vi "Begin.vi"() -> (0 "Error out":errorcluster)   [LabVIEW 2015]
doc: "Called before other user functions, this VI is expected to open initial I/O refnums, load in file data, and do all program initialization. Notice that the <B>error out</B> terminal is simply used for data flow. Wiring it to other structures or subVIs ensures that this VI runs first."
uses:
  <vilib>/Rock Robotics/WPI/Joystick/WPI_JoystickDeviceEnum.ctl
  <vilib>/Rock Robotics/WPI/Solenoid/WPI_SolenoidChannel.ctl
  <vilib>/Rock Robotics/WPI/CAN/TalonSRX/WPI_CANTalonSRX_APIControlMode.ctl
  <vilib>/Rock Robotics/SystemInterfaces/DIO/FPGA_DIOPWMChannel.ctl
  <vilib>/Rock Robotics/SystemInterfaces/AI/FPGA_AIGyroChannel.ctl
  <vilib>/Rock Robotics/SystemInterfaces/DIO/FPGA_DIOChannel.ctl
  <vilib>/Rock Robotics/WPI/CAN/TalonSRX/WPI_CANTalonSRX_APIFeedbackSelect.ctl
  <vilib>/Rock Robotics/WPI/Solenoid/WPI_SolenoidValue.ctl
  <vilib>/Rock Robotics/SystemInterfaces/i2clib/i2c_bus.ctl
  <vilib>/Rock Robotics/WPI/MotorControl/WPI_MotorControlOpenCANTalonSRX.vi
  <vilib>/Rock Robotics/WPI/Solenoid/WPI_SolenoidOpenDouble.vi
  <vilib>/Rock Robotics/WPI/Gyro/WPI_GyroAnalogOpen.vi
  <vilib>/Rock Robotics/WPI/Switch/WPI_SwitchOpenLimit.vi
  <vilib>/Rock Robotics/WPI/MotorControl/WPI_MotorControlOpen VictorSP.vi
  Global Variables/Temp Variables.vi
  <vilib>/Rock Robotics/WPI/Solenoid/WPI_SolenoidOpenSingle.vi
  <vilib>/Rock Robotics/WPI/Solenoid/WPI_SolenoidSetEnum.vi
  Global Variables/refnum names.vi
  Global Variables/Calibrations.vi
  <vilib>/Rock Robotics/SystemInterfaces/AI/FPGA_AIChannel.ctl
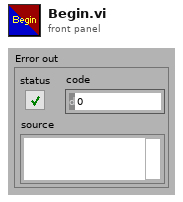
[diagram p1: front panel]
types:
  T1 = typedef "i2c_bus.ctl" = enum16{"I2C On-Board", "I2C MXP", "Invalid"}
  T2 = enum8{"ConfigMode", "AccOnly", "MagOnly", "GyroOnly", "AccMag", "AccGyro", "MagGyro", "AMG", "IMU", "Compass", "M4G", "NDOF_FMC_OFF", "NDOF"}
  T3 = enum32{"P0", "P1", "P2", "P3", "P4", "P5", "P6", "P7"}
  T4 = typedef "WPI_SolenoidChannel.ctl" = enum8{"Solenoid 0", "Solenoid 1", "Solenoid 2", "Solenoid 3", "Solenoid 4", "Solenoid 5", "Solenoid 6", "Solenoid 7", "Invalid"}
  T5 = typedef "WPI_SolenoidValue.ctl" = enum16{"Off", "On", "Forward", "Reverse"}
  T6 = typedef "WPI_CANTalonSRX_APIControlMode.ctl" = enum8{"Percent VBus", "Speed", "Position", "Slave", "Unchanged / Invalid", "Voltage Compensation", "Current", "Motion Profile"}
  T7 = typedef "FPGA_DIOChannel.ctl" = enum8{"DIO 0", "DIO 1", "DIO 2", "DIO 3", "DIO 4", "DIO 5", "DIO 6", "DIO 7", "DIO 8", "DIO 9", "DIO MXP 0", "DIO MXP 1", "DIO MXP 2", "DIO MXP 3", "DIO MXP 4", "DIO MXP 5", "DIO MXP 6", "DIO MXP 7", "DIO MXP 8", "DIO MXP 9", "DIO MXP 10", "DIO MXP 11", "DIO MXP 12", "DIO MXP 13", "DIO MXP 14", "DIO MXP 15", "Invalid"}
  T8 = typedef "WPI_JoystickDeviceEnum.ctl" = enum16{"USB 0", "USB 1", "USB 2", "USB 3", "USB 4", "USB 5"}
  T9 = typedef "WPI_CANTalonSRX_APIFeedbackSelect.ctl" = enum16{"Digital Quadrature Encoder", "Analog Potentiometer", "Analog Encoder", "Count on Quad-A (Rising-Edge)", "Count on Quad-A (Falling-Edge)", "CTR Magnetic Enc (Absolute)", "CTR Magnetic Enc (Relative)", "Pulse Width"}
  T10 = typedef "FPGA_AIGyroChannel.ctl" = enum8{"AI 0", "AI 1", "Invalid"}
  T11 = typedef "FPGA_DIOPWMChannel.ctl" = enum8{"PWM 0", "PWM 1", "PWM 2", "PWM 3", "PWM 4", "PWM 5", "PWM 6", "PWM 7", "PWM 8", "PWM 9", "PWM MXP 0", "PWM MXP 1", "PWM MXP 2", "PWM MXP 3", "PWM MXP 4", "PWM MXP 5", "PWM MXP 6", "PWM MXP 7", "PWM MXP 8", "PWM MXP 9", "Invalid"}
  T12 = typedef "FPGA_AIChannel.ctl" = enum8{"AI 0", "AI 1", "AI 2", "AI 3", "AI MXP 0", "AI MXP 1", "AI MXP 2", "AI MXP 3", "Invalid"}
  T13 = typedef "WPI_MotorControlDeviceRef.ctl" = cluster{"DeviceStatus":errorcluster, "Type":T14, "PWM":cluster{"PWM Channel":T11, "DeadBand":T15}, "CAN":cluster{"Device Number":u8, "Control Mode":T16, "Semaphore":T17, "Max Vout":dbl, "TalonSRX Control Mode":T6}, "Invert":bool}
  T14 = typedef "WPI_MotorControlType.ctl" = enum16{"PWM", "CAN", "CANTalonSRX"}
  T15 = typedef "WPI_PWMDeadband.ctl" = cluster{"Name":string, "maxPositivePwm":i32, "minPositivePwm":i32, "centerPwm":i32, "maxNegativePwm":i32, "minNegativePwm":i32, "angularRange":u16}
  T16 = typedef "WPI_CANJaguar_ControlMode.ctl" = enum8{"Percent VBus", "Current", "Speed", "Position", "Voltage"}
  T17 = typedef "Semaphore RefNum" = refnum<k1>
  T18 = typedef "WPI_I2CDevRef.ctl" = cluster{"DevStatus":errorcluster, "Device Address":u8, "Handle":i32, "I2C Bus":T1}
  T19 = typedef "WPI_PotentiometerDevRef.ctl" = cluster{"DevStatus":errorcluster, "Analog Channel":T12, "Invert Output":bool}
  T20 = typedef "WPI_SolenoidDevRef.ctl" = cluster{"DevStatus":errorcluster, "Pneumatics Control Module":u8, "Forward Solenoid Channel":T4, "Reverse Solenoid Channel":T4}
  T21 = typedef "WPI_GyroDevRef.ctl" = cluster{"DevStatus":errorcluster, "Analog Channel":T12, "Offset":dbl, "Gain (VoltsPerDegree/Second)":dbl, "Gyro Type":enum16{"Analog", "XRS450"}, "Handle":i32, "SPI Bus":T22, "Device Found":bool, "Sample Rate":dbl, "Calibrate On Open":bool}
  T22 = typedef "spi_bus.ctl" = enum16{"SPI On-Board, CS0", "SPI On-Board, CS1", "SPI On-Board, CS2", "SPI On-Board, CS3", "SPI MXP", "Invalid"}
  T23 = typedef "WPI_SwitchDevRef.ctl" = cluster{"DevStatus":errorcluster, "DIO Channel":T7, "CntIndex":T24, "Normally Closed":bool}
  T24 = typedef "FPGA_CounterCtrSystemIndex.ctl" = enum8{"Ctr 0", "Ctr 1", "Ctr 2", "Ctr 3", "Ctr 4", "Ctr 5", "Ctr 6", "Ctr 7", "Invalid"}
  T25 = typedef "WPI_DigitalInputDevRef.ctl" = cluster{"DevStatus":errorcluster, "DIO Channel":T7}
  T26 = typedef "WPI_JoystickDevRef.ctl" = cluster{"Device":T8}
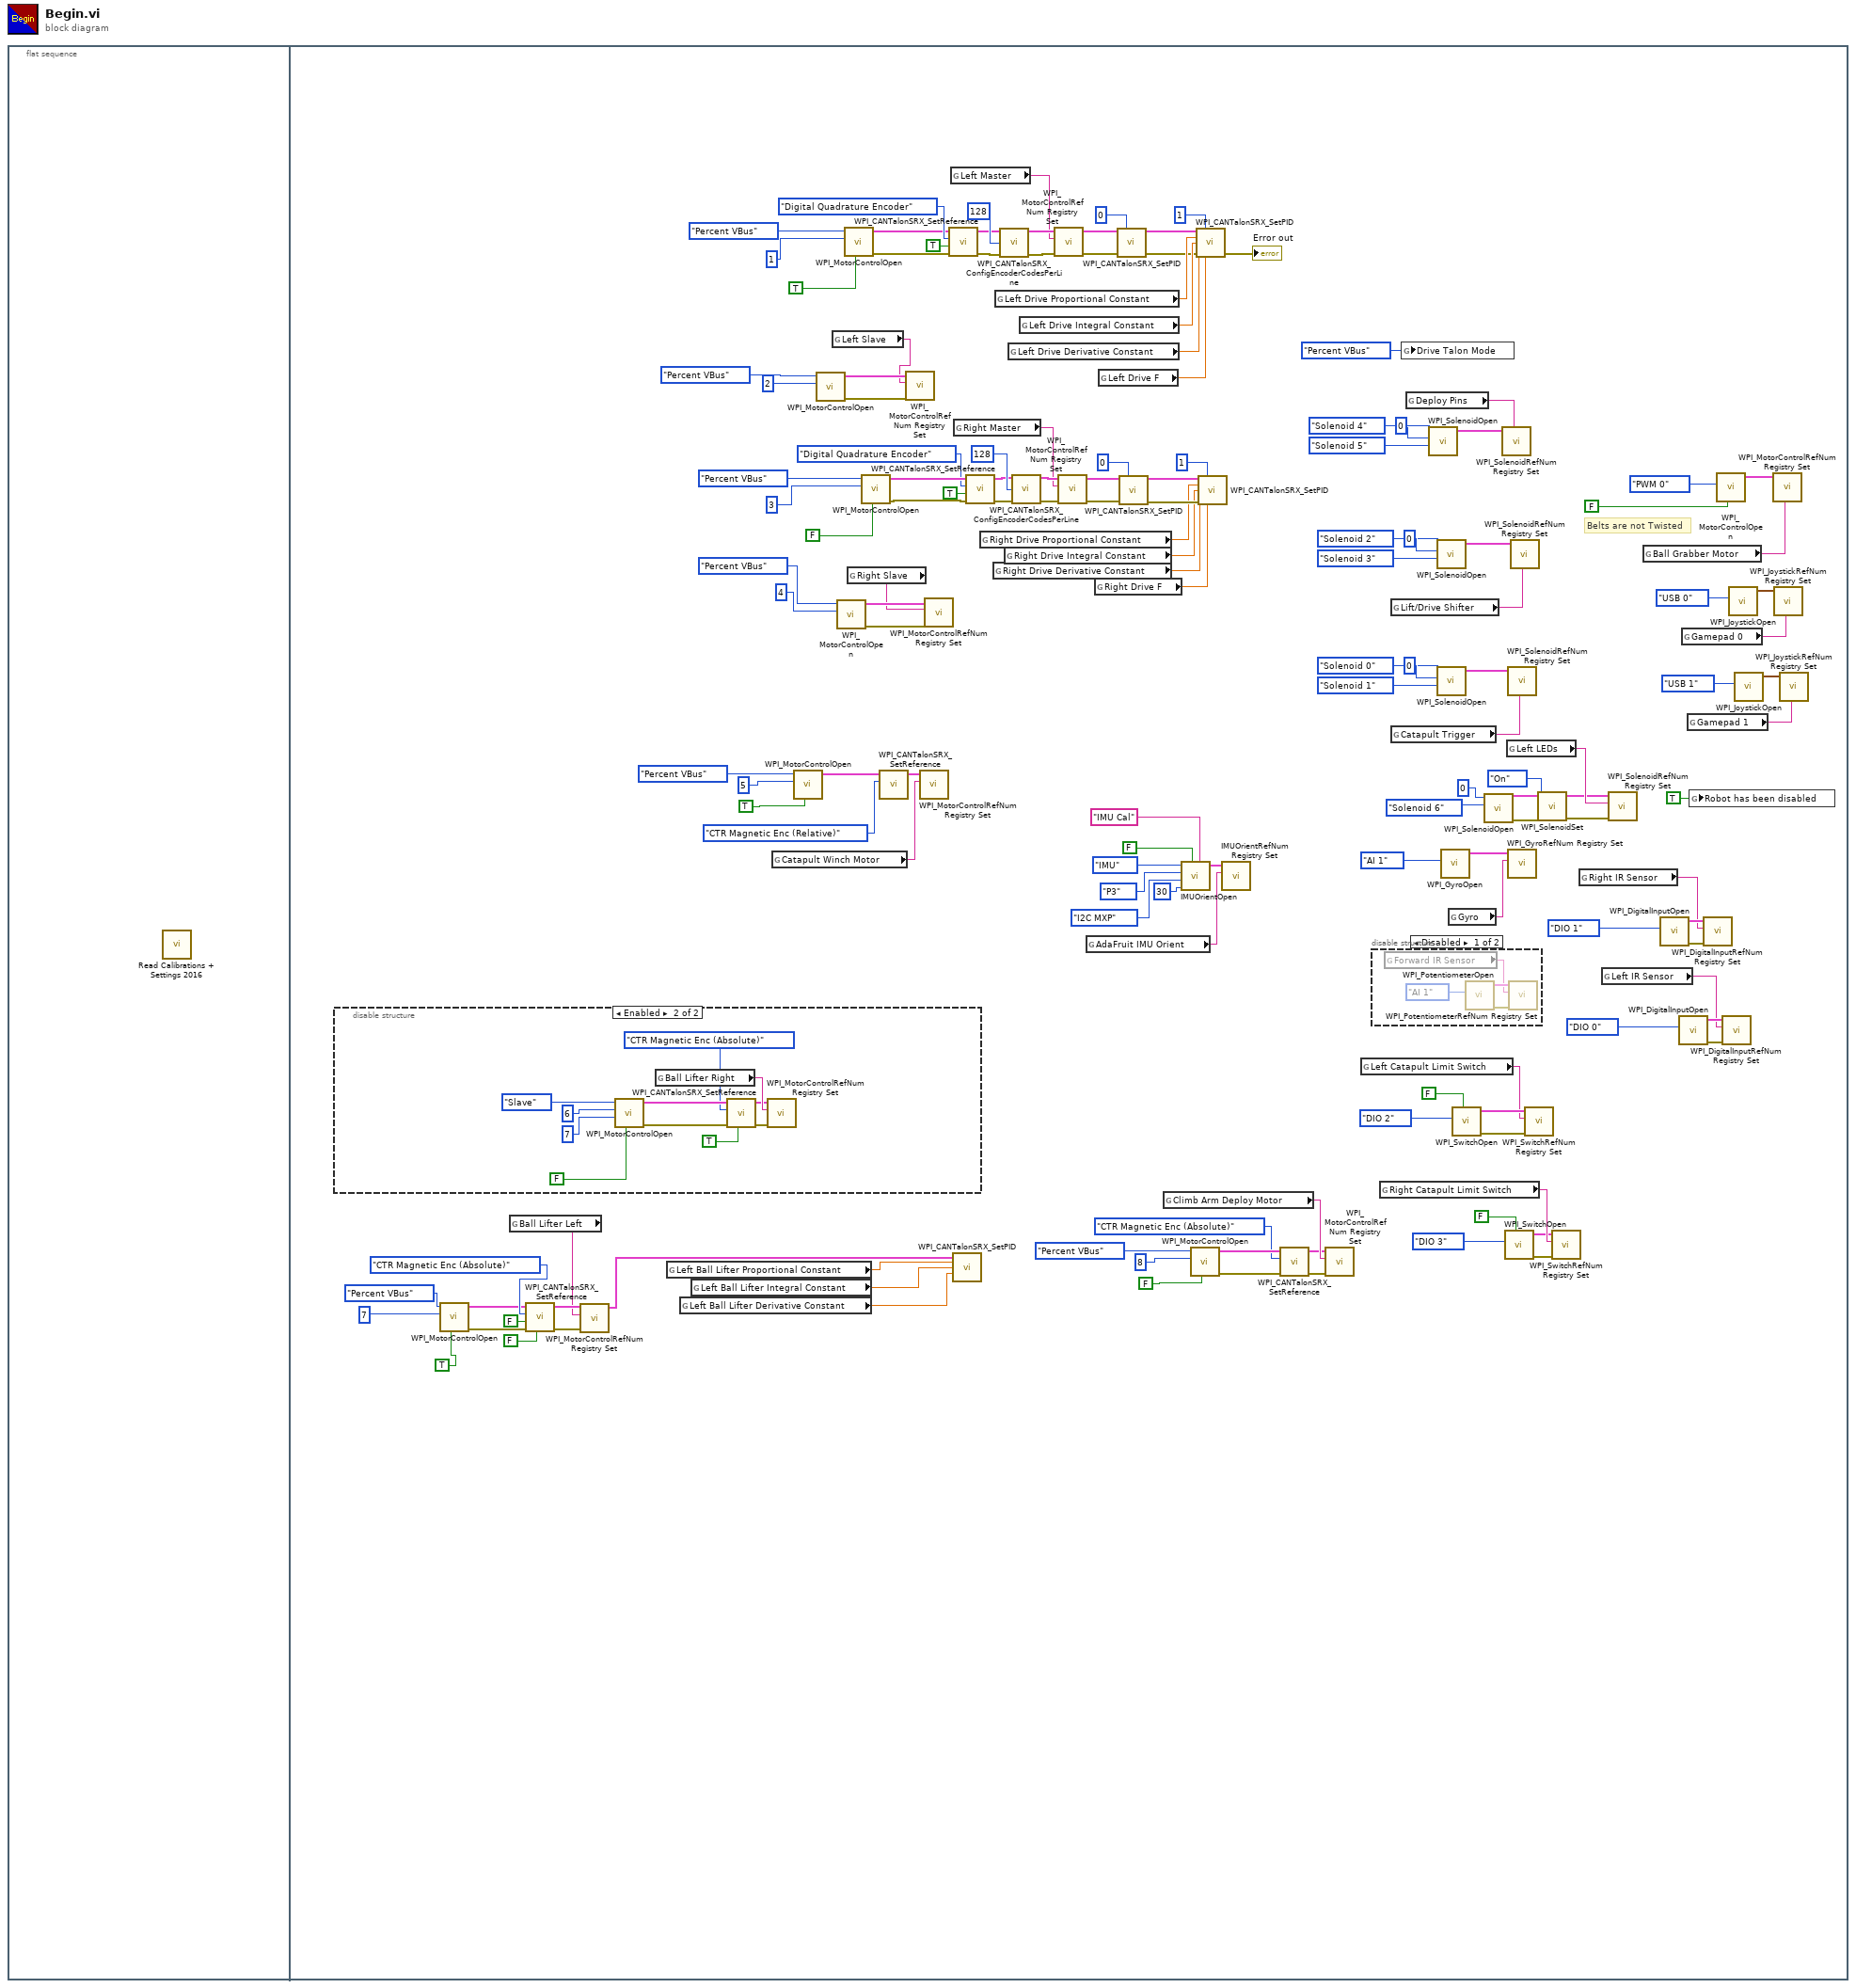
[diagram p0: block diagram]
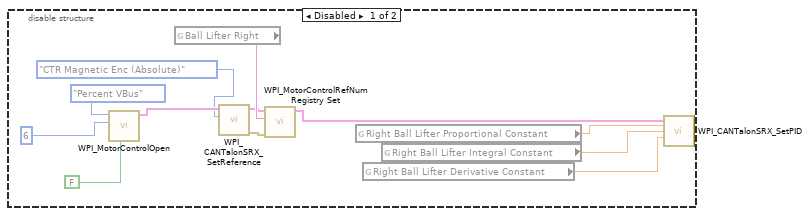
[diagram p3: hidden frame]
diagram:
  n1 = flat-sequence {
    frame #0 {
      n2 = call "Read Calibrations + Settings 2016.vi"() -> ()  [unwired: 12 in]
    }
    frame #1 {
      # "Belts are not Twisted"
      n3 = disable-structure shown="Enabled" {
        frame Disabled {
          n4 = call-poly <vilib>:"WPI_MotorControlOpen.vi"("Invert"=FALSE, "Device Number"=u8 6, "Control Mode"=WPI_CANTalonSRX_APIControlMode."Percent VBus") -> ("MotorControlDeviceRef"=w161:T13)  [unwired: 7 in, 1 out]
          n5 = global read "refnum names.vi" "Ball Lifter Right"() -> (w166:string)
          n6 = call <vilib>:"WPI_CANTalonSRX_SetReference.vi"("Feedback Reference"=WPI_CANTalonSRX_APIFeedbackSelect."CTR Magnetic Enc (Absolute)", "CAN Talon SRX Ref"=w161) -> ("error out"=w162:errorcluster, "CAN Talon SRX Ref"=w160:T13)  [unwired: 8 in]
          n7 = call <vilib>:"WPI_MotorControlRefNum Registry Set.vi"("error in (no error)"=w162, "refnum name"=w166, "MotorControlDevRef"=w160) -> ("MotorControlDevRef"=w155:T13)  [unwired: 7 in, 1 out]
          n8 = global read "Calibrations.vi" "Right Ball Lifter Proportional Constant"() -> (w158:dbl)
          n9 = global read "Calibrations.vi" "Right Ball Lifter Derivative Constant"() -> (w156:dbl)
          n10 = global read "Calibrations.vi" "Right Ball Lifter Integral Constant"() -> (w157:dbl)
          n11 = call <vilib>:"WPI_CANTalonSRX_SetPID.vi"("CAN Talon SRX Ref"=w155, "P"=w158, "I"=w157, "D"=w156) -> ()  [unwired: 10 in, 2 out]
        }
        frame Enabled {
          n12 = call-poly <vilib>:"WPI_MotorControlOpen.vi"("Invert"=FALSE, "Master Device Number"=u8 7, "Device Number"=u8 6, "Control Mode"=WPI_CANTalonSRX_APIControlMode."Slave") -> ("error out"=w174:errorcluster, "MotorControlDeviceRef"=w173:T13)  [unwired: 6 in]
          n13 = global read "refnum names.vi" "Ball Lifter Right"() -> (w177:string)
          n14 = call <vilib>:"WPI_CANTalonSRX_SetReference.vi"("Reverse Closed-Loop Output"=TRUE, "error in (no error)"=w174, "Feedback Reference"=WPI_CANTalonSRX_APIFeedbackSelect."CTR Magnetic Enc (Absolute)", "CAN Talon SRX Ref"=w173) -> ("error out"=w175:errorcluster, "CAN Talon SRX Ref"=w176:T13)  [unwired: 6 in]
          n15 = call <vilib>:"WPI_MotorControlRefNum Registry Set.vi"("error in (no error)"=w175, "refnum name"=w177, "MotorControlDevRef"=w176) -> ()  [unwired: 7 in, 2 out]
        }
      }
      n16 = call-poly <vilib>:"WPI_MotorControlOpen.vi"("Invert"=TRUE, "Device Number"=u8 7, "Control Mode"=WPI_CANTalonSRX_APIControlMode."Percent VBus") -> ("error out"=w75:errorcluster, "MotorControlDeviceRef"=w74:T13)  [unwired: 7 in]
      n17 = global read "refnum names.vi" "Ball Lifter Left"() -> (w44:string)
      n18 = call <vilib>:"WPI_CANTalonSRX_SetReference.vi"("Reverse Closed-Loop Output"=FALSE, "error in (no error)"=w75, "Reverse Feedback Sensor"=FALSE, "Feedback Reference"=WPI_CANTalonSRX_APIFeedbackSelect."CTR Magnetic Enc (Absolute)", "CAN Talon SRX Ref"=w74) -> ("error out"=w72:errorcluster, "CAN Talon SRX Ref"=w73:T13)  [unwired: 5 in]
      n19 = call <vilib>:"WPI_MotorControlRefNum Registry Set.vi"("error in (no error)"=w72, "refnum name"=w44, "MotorControlDevRef"=w73) -> ("MotorControlDevRef"=w150:T13)  [unwired: 7 in, 1 out]
      n20 = global read "Calibrations.vi" "Left Ball Lifter Proportional Constant"() -> (w108:dbl)
      n21 = global read "Calibrations.vi" "Left Ball Lifter Derivative Constant"() -> (w106:dbl)
      n22 = global read "Calibrations.vi" "Left Ball Lifter Integral Constant"() -> (w107:dbl)
      n23 = global read "refnum names.vi" "Catapult Winch Motor"() -> (w37:string)
      n24 = call-poly <vilib>:"WPI_MotorControlOpen.vi"("Invert"=TRUE, "Device Number"=u8 5, "Control Mode"=WPI_CANTalonSRX_APIControlMode."Percent VBus") -> ("MotorControlDeviceRef"=w69:T13)  [unwired: 7 in, 1 out]
      n25 = call-poly <vilib>:"WPI_MotorControlOpen.vi"("Device Number"=u8 2, "Control Mode"=WPI_CANTalonSRX_APIControlMode."Percent VBus") -> ("error out"=w20:errorcluster, "MotorControlDeviceRef"=w21:T13)  [unwired: 8 in]
      n26 = global read "refnum names.vi" "Left Slave"() -> (w19:string)
      n27 = call-poly <vilib>:"WPI_MotorControlOpen.vi"("Device Number"=u8 4, "Control Mode"=WPI_CANTalonSRX_APIControlMode."Percent VBus") -> ("error out"=w17:errorcluster, "MotorControlDeviceRef"=w18:T13)  [unwired: 8 in]
      n28 = call-poly <vilib>:"WPI_MotorControlOpen.vi"("Invert"=TRUE, "Device Number"=u8 1, "Control Mode"=WPI_CANTalonSRX_APIControlMode."Percent VBus") -> ("error out"=w67:errorcluster, "MotorControlDeviceRef"=w65:T13)  [unwired: 7 in]
      n29 = global read "refnum names.vi" "Right Slave"() -> (w16:string)
      n30 = call-poly <vilib>:"WPI_MotorControlOpen.vi"("Invert"=FALSE, "Device Number"=u8 3, "Control Mode"=WPI_CANTalonSRX_APIControlMode."Percent VBus") -> ("error out"=w10:errorcluster, "MotorControlDeviceRef"=w63:T13)  [unwired: 7 in]
      n31 = call <vilib>:"WPI_CANTalonSRX_SetReference.vi"("Feedback Reference"=WPI_CANTalonSRX_APIFeedbackSelect."CTR Magnetic Enc (Relative)", "CAN Talon SRX Ref"=w69) -> ("CAN Talon SRX Ref"=w70:T13)  [unwired: 8 in, 1 out]
      n32 = call <vilib>:"WPI_MotorControlRefNum Registry Set.vi"("error in (no error)"=w20, "refnum name"=w19, "MotorControlDevRef"=w21) -> ()  [unwired: 7 in, 2 out]
      n33 = call <vilib>:"WPI_MotorControlRefNum Registry Set.vi"("refnum name"=w37, "MotorControlDevRef"=w70) -> ()  [unwired: 8 in, 2 out]
      n34 = call <vilib>:"WPI_MotorControlRefNum Registry Set.vi"("error in (no error)"=w17, "refnum name"=w16, "MotorControlDevRef"=w18) -> ()  [unwired: 7 in, 2 out]
      n35 = call <vilib>:"WPI_CANTalonSRX_SetReference.vi"("error in (no error)"=w67, "Reverse Feedback Sensor"=TRUE, "Feedback Reference"=WPI_CANTalonSRX_APIFeedbackSelect."Digital Quadrature Encoder", "CAN Talon SRX Ref"=w65) -> ("error out"=w120:errorcluster, "CAN Talon SRX Ref"=w121:T13)  [unwired: 6 in]
      n36 = global read "refnum names.vi" "Left Master"() -> (w29:string)
      n37 = call <vilib>:"WPI_CANTalonSRX_SetPID.vi"("CAN Talon SRX Ref"=w150, "P"=w108, "I"=w107, "D"=w106) -> ()  [unwired: 10 in, 2 out]
      n38 = global read "refnum names.vi" "Right Master"() -> (w64:string)
      n39 = call <vilib>:"WPI_CANTalonSRX_SetReference.vi"("error in (no error)"=w10, "Reverse Feedback Sensor"=TRUE, "Feedback Reference"=WPI_CANTalonSRX_APIFeedbackSelect."Digital Quadrature Encoder", "CAN Talon SRX Ref"=w63) -> ("error out"=w127:errorcluster, "CAN Talon SRX Ref"=w125:T13)  [unwired: 6 in]
      n40 = global read "Calibrations.vi" "Right Drive Proportional Constant"() -> (w135:dbl)
      n41 = global read "Calibrations.vi" "Right Drive Derivative Constant"() -> (w137:dbl)
      n42 = global read "Calibrations.vi" "Left Drive Proportional Constant"() -> (w130:dbl)
      n43 = call <vilib>:"WPI_CANTalonSRX_ConfigEncoderCodesPerLine.vi"("CAN Talon SRX Ref"=w121, "Number Encoder Lines\n(Counts Per Rotation)"=u32 128 ("Number Encoder Lines\n(Counts Per Rotation)"), "error in (no error)"=w120) -> ("CAN Talon SRX Ref"=w122:T13, "error out"=w139:errorcluster)  [unwired: 11 in]
      n44 = global read "Calibrations.vi" "Right Drive Integral Constant"() -> (w136:dbl)
      n45 = global read "Calibrations.vi" "Left Drive Derivative Constant"() -> (w132:dbl)
      n46 = call <vilib>:"WPI_CANTalonSRX_ConfigEncoderCodesPerLine.vi"("CAN Talon SRX Ref"=w125, "Number Encoder Lines\n(Counts Per Rotation)"=u32 128 ("Number Encoder Lines\n(Counts Per Rotation)"), "error in (no error)"=w127) -> ("CAN Talon SRX Ref"=w126:T13, "error out"=w124:errorcluster)  [unwired: 11 in]
      n47 = global read "Calibrations.vi" "Left Drive Integral Constant"() -> (w131:dbl)
      n48 = call <vilib>:"WPI_MotorControlRefNum Registry Set.vi"("error in (no error)"=w139, "refnum name"=w29, "MotorControlDevRef"=w122) -> ("error out"=→"Error out":errorcluster, "MotorControlDevRef"=w113:T13)  [unwired: 7 in]
      n49 = call <vilib>:"WPI_MotorControlRefNum Registry Set.vi"("error in (no error)"=w124, "refnum name"=w64, "MotorControlDevRef"=w126) -> ("error out"=w140:errorcluster, "MotorControlDevRef"=w117:T13)  [unwired: 7 in]
      n50 = global read "refnum names.vi" "AdaFruit IMU Orient"() -> (w1:string)
      n51 = global read "Calibrations.vi" "Right Drive F"() -> (w138:dbl)
      n52 = global read "Calibrations.vi" "Left Drive F"() -> (w133:dbl)
      n53 = call <vilib>:"WPI_CANTalonSRX_SetPID.vi"("CAN Talon SRX Ref"=w113, "Parameter Slot"=u8 0) -> ("CAN Talon SRX Ref"=w119:T13)  [unwired: 12 in, 1 out]
      n54 = call <vilib>:"WPI_CANTalonSRX_SetPID.vi"("CAN Talon SRX Ref"=w117, "Parameter Slot"=u8 0, "error in (no error)"=w140) -> ("CAN Talon SRX Ref"=w116:T13, "error out"=w141:errorcluster)  [unwired: 11 in]
      n55 = global read "refnum names.vi" "Climb Arm Deploy Motor"() -> (w85:string)
      n56 = call "IMUOrientOpen.vi"("Stored Cal File"="IMU Cal", "Calibrate?"=FALSE, "Status delay"=30, "I2C Bus"=i2c_bus."I2C MXP", "Placement"=T3."P3", "Op Mode"=T2."IMU") -> ("I2CDevRef"=w6:T18)  [unwired: 2 in, 3 out]
      n57 = call-poly <vilib>:"WPI_MotorControlOpen.vi"("Invert"=FALSE, "Device Number"=u8 8, "Control Mode"=WPI_CANTalonSRX_APIControlMode."Percent VBus") -> ("error out"=w78:errorcluster, "MotorControlDeviceRef"=w79:T13)  [unwired: 7 in]
      n58 = call <vilib>:"WPI_CANTalonSRX_SetPID.vi"("CAN Talon SRX Ref"=w119, "Parameter Slot"=u8 1, "P"=w130, "I"=w131, "D"=w132, "F"=w133) -> ()  [unwired: 8 in, 2 out]
      n59 = call <vilib>:"WPI_CANTalonSRX_SetPID.vi"("CAN Talon SRX Ref"=w116, "Parameter Slot"=u8 1, "P"=w135, "I"=w136, "D"=w137, "error in (no error)"=w141, "F"=w138) -> ()  [unwired: 7 in, 2 out]
      n60 = call "IMUOrientRefNum Registry Set.vi"("refnum name"=w1, "I2CDevRef in"=w6) -> ()  [unwired: 8 in, 2 out]
      n61 = call <vilib>:"WPI_CANTalonSRX_SetReference.vi"("error in (no error)"=w78, "Feedback Reference"=WPI_CANTalonSRX_APIFeedbackSelect."CTR Magnetic Enc (Absolute)", "CAN Talon SRX Ref"=w79) -> ("error out"=w81:errorcluster, "CAN Talon SRX Ref"=w80:T13)  [unwired: 7 in]
      n62 = call <vilib>:"WPI_MotorControlRefNum Registry Set.vi"("error in (no error)"=w81, "refnum name"=w85, "MotorControlDevRef"=w80) -> ()  [unwired: 7 in, 2 out]
      n63 = global read "refnum names.vi" "Left Catapult Limit Switch"() -> (w61:string)
      n64 = disable-structure shown="Disabled" {
        frame Disabled {
          n65 = global read "refnum names.vi" "Forward IR Sensor"() -> (w152:string)
          n66 = call <vilib>:"WPI_PotentiometerOpen.vi"("Analog Channel"=FPGA_AIChannel."AI 1") -> ("error out"=w154:errorcluster, "PotDevRef"=w153:T19)  [unwired: 9 in]
          n67 = call <vilib>:"WPI_PotentiometerRefNum Registry Set.vi"("error in (no error)"=w154, "refnum name"=w152, "PotDevRef"=w153) -> ()  [unwired: 7 in, 2 out]
        }
        frame Enabled {
        }
      }
      n68 = global read "refnum names.vi" "Right Catapult Limit Switch"() -> (w105:string)
      n69 = global read "refnum names.vi" "Lift/Drive Shifter"() -> (w90:string)
      n70 = global read "refnum names.vi" "Catapult Trigger"() -> (w43:string)
      n71 = global write "Temp Variables.vi" "Drive Talon Mode"(WPI_CANTalonSRX_APIControlMode."Percent VBus" ("Drive Talon Mode")) -> ()
      n72 = global read "refnum names.vi" "Deploy Pins"() -> (w11:string)
      n73 = call-poly <vilib>:"WPI_SolenoidOpen.vi"("Reverse Solenoid Channel"=WPI_SolenoidChannel."Solenoid 5", "Forward Solenoid Channel"=WPI_SolenoidChannel."Solenoid 4", "Pneumatics Control Module (0)"=u8 0) -> ("SolenoidDevRef"=w12:T20)  [unwired: 7 in, 1 out]
      n74 = call-poly <vilib>:"WPI_SolenoidOpen.vi"("Reverse Solenoid Channel"=WPI_SolenoidChannel."Solenoid 3", "Forward Solenoid Channel"=WPI_SolenoidChannel."Solenoid 2", "Pneumatics Control Module (0)"=u8 0) -> ("SolenoidDevRef"=w89:T20)  [unwired: 7 in, 1 out]
      n75 = call-poly <vilib>:"WPI_SolenoidOpen.vi"("Reverse Solenoid Channel"=WPI_SolenoidChannel."Solenoid 1", "Forward Solenoid Channel"=WPI_SolenoidChannel."Solenoid 0", "Pneumatics Control Module (0)"=u8 0) -> ("SolenoidDevRef"=w42:T20)  [unwired: 7 in, 1 out]
      n76 = call-poly <vilib>:"WPI_GyroOpen.vi"("Analog Channel"=FPGA_AIGyroChannel."AI 1") -> ("GyroDevRef"=w51:T21)  [unwired: 8 in, 2 out]
      n77 = global read "refnum names.vi" "Gyro"() -> (w2:string)
      n78 = call-poly <vilib>:"WPI_SwitchOpen.vi"("Normally Closed"=FALSE, "DIO Channel"=FPGA_DIOChannel."DIO 2") -> ("error out"=w98:errorcluster, "SwitchDevRef"=w97:T23)  [unwired: 8 in]
      n79 = call-poly <vilib>:"WPI_SolenoidOpen.vi"("Solenoid Channel"=WPI_SolenoidChannel."Solenoid 6", "Pneumatics Control Module (0)"=u8 0) -> ("error out"=w146:errorcluster, "SolenoidDevRef"=w144:T20)  [unwired: 8 in]
      n80 = call <vilib>:"WPI_SolenoidRefNum Registry Set.vi"("refnum name"=w11, "SolenoidDevRef"=w12) -> ()  [unwired: 8 in, 2 out]
      n81 = call-poly <vilib>:"WPI_SwitchOpen.vi"("Normally Closed"=FALSE, "DIO Channel"=FPGA_DIOChannel."DIO 3") -> ("error out"=w101:errorcluster, "SwitchDevRef"=w102:T23)  [unwired: 8 in]
      n82 = global read "refnum names.vi" "Left LEDs"() -> (w149:string)
      n83 = call <vilib>:"WPI_SolenoidRefNum Registry Set.vi"("refnum name"=w43, "SolenoidDevRef"=w42) -> ()  [unwired: 8 in, 2 out]
      n84 = call <vilib>:"WPI_GyroRefNum Registry Set.vi"("refnum name"=w2, "GyroDevRef"=w51) -> ()  [unwired: 8 in, 2 out]
      n85 = call <vilib>:"WPI_SolenoidRefNum Registry Set.vi"("refnum name"=w90, "SolenoidDevRef"=w89) -> ()  [unwired: 8 in, 2 out]
      n86 = call <vilib>:"WPI_SwitchRefNum Registry Set.vi"("error in (no error)"=w98, "refnum name"=w61, "SwitchDevRef"=w97) -> ()  [unwired: 7 in, 2 out]
      n87 = call-poly <vilib>:"WPI_SolenoidSet.vi"("error in (no error)"=w146, "Value"=WPI_SolenoidValue."On", "SolenoidDevRef"=w144) -> ("error out"=w148:errorcluster, "SolenoidDevRef"=w147:T20)  [unwired: 7 in]
      n88 = call <vilib>:"WPI_SwitchRefNum Registry Set.vi"("error in (no error)"=w101, "refnum name"=w105, "SwitchDevRef"=w102) -> ()  [unwired: 7 in, 2 out]
      n89 = global read "refnum names.vi" "Right IR Sensor"() -> (w59:string)
      n90 = global read "refnum names.vi" "Left IR Sensor"() -> (w55:string)
      n91 = call <vilib>:"WPI_SolenoidRefNum Registry Set.vi"("error in (no error)"=w148, "refnum name"=w149, "SolenoidDevRef"=w147) -> ()  [unwired: 7 in, 2 out]
      n92 = global read "refnum names.vi" "Ball Grabber Motor"() -> (w50:string)
      n93 = call <vilib>:"WPI_DigitalInputOpen.vi"("DIO Channel"=FPGA_DIOChannel."DIO 1") -> ("error out"=w57:errorcluster, "DigitalInputDevRef"=w60:T25)  [unwired: 9 in]
      n94 = call <vilib>:"WPI_DigitalInputOpen.vi"("DIO Channel"=FPGA_DIOChannel."DIO 0") -> ("error out"=w53:errorcluster, "DigitalInputDevRef"=w56:T25)  [unwired: 9 in]
      n95 = global read "refnum names.vi" "Gamepad 0"() -> (w28:string)
      n96 = global read "refnum names.vi" "Gamepad 1"() -> (w91:string)
      n97 = global write "Temp Variables.vi" "Robot has been disabled"(TRUE ("Robot has been disabled")) -> ()
      n98 = call <vilib>:"WPI_DigitalInputRefNum Registry Set.vi"("error in (no error)"=w57, "refnum name"=w59, "DigitalInputDevRef"=w60) -> ()  [unwired: 7 in, 2 out]
      n99 = call-poly <vilib>:"WPI_MotorControlOpen.vi"("Invert"=FALSE, "PWM Channel"=FPGA_DIOPWMChannel."PWM 0") -> ("MotorControlDeviceRef"=w49:T13)  [unwired: 8 in, 1 out]
      n100 = call <vilib>:"WPI_DigitalInputRefNum Registry Set.vi"("error in (no error)"=w53, "refnum name"=w55, "DigitalInputDevRef"=w56) -> ()  [unwired: 7 in, 2 out]
      n101 = call <vilib>:"WPI_JoystickOpen.vi"("JoystickDevice"=WPI_JoystickDeviceEnum."USB 0") -> ("JoystickDevRef"=w27:T26)  [unwired: 10 in]
      n102 = call <vilib>:"WPI_JoystickOpen.vi"("JoystickDevice"=WPI_JoystickDeviceEnum."USB 1") -> ("JoystickDevRef"=w92:T26)  [unwired: 10 in]
      n103 = call <vilib>:"WPI_MotorControlRefNum Registry Set.vi"("refnum name"=w50, "MotorControlDevRef"=w49) -> ()  [unwired: 8 in, 2 out]
      n104 = call <vilib>:"WPI_JoystickRefNum Registry Set.vi"("refnum name"=w28, "JoystickDevRef"=w27) -> ()  [unwired: 8 in, 2 out]
      n105 = call <vilib>:"WPI_JoystickRefNum Registry Set.vi"("refnum name"=w91, "JoystickDevRef"=w92) -> ()  [unwired: 8 in, 2 out]
    }
  }
